vi "AMC QMH Template.vi"() -> ()   [LabVIEW 2017]
panel:
  out "Status":string
  in  "Process":bool
  in  "Exit":bool
  in  "State Variables":cluster{"CurrentFile":path}
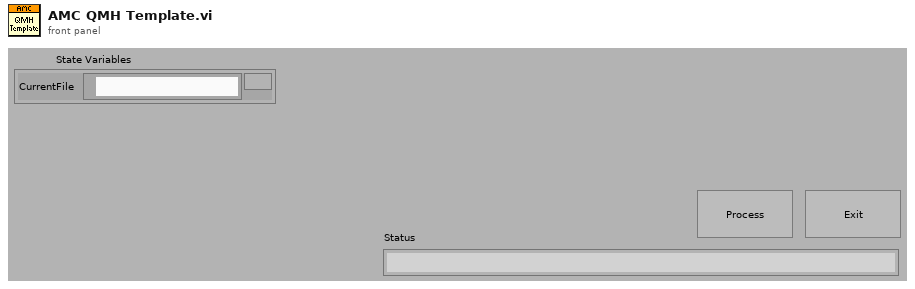
[diagram p1: front panel]
types:
  T1 = typedef "amc_Message Queue.ctl" = refnum<queue>
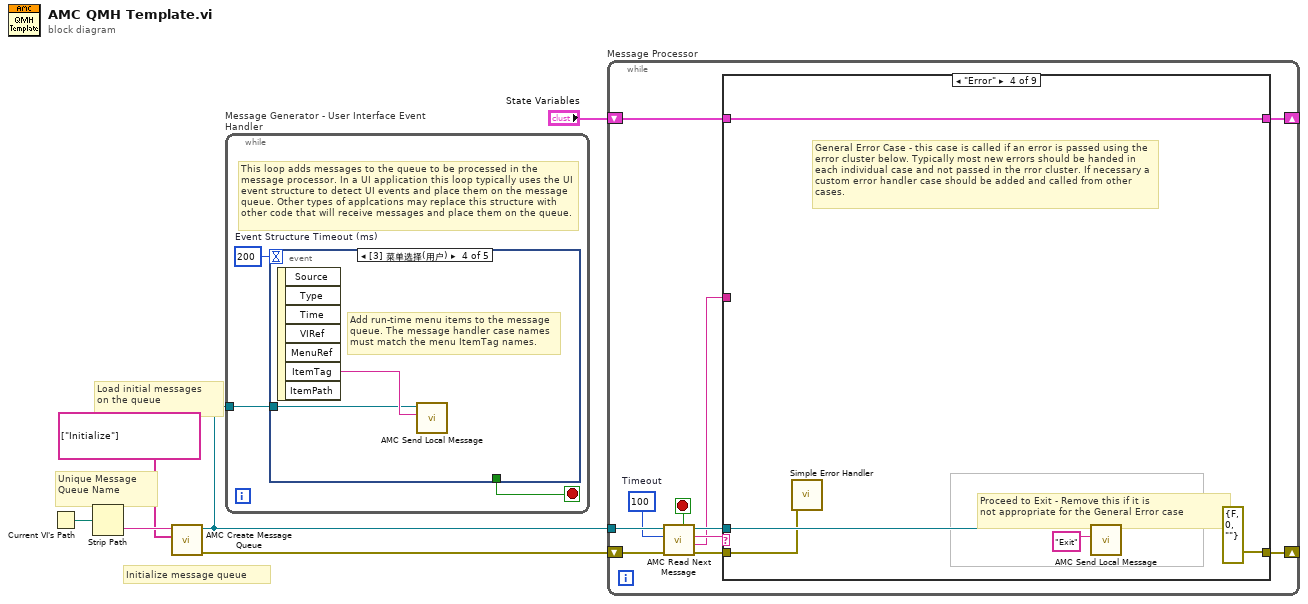
[diagram p0: block diagram]
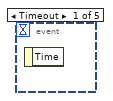
[diagram p2: hidden frame]
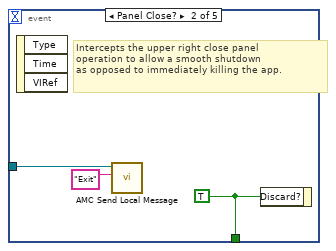
[diagram p3: hidden frame]
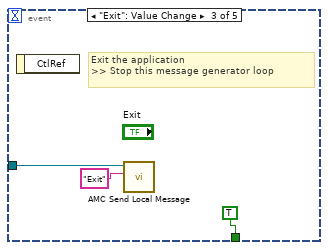
[diagram p4: hidden frame]
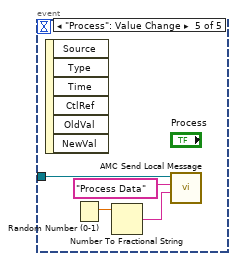
[diagram p5: hidden frame]
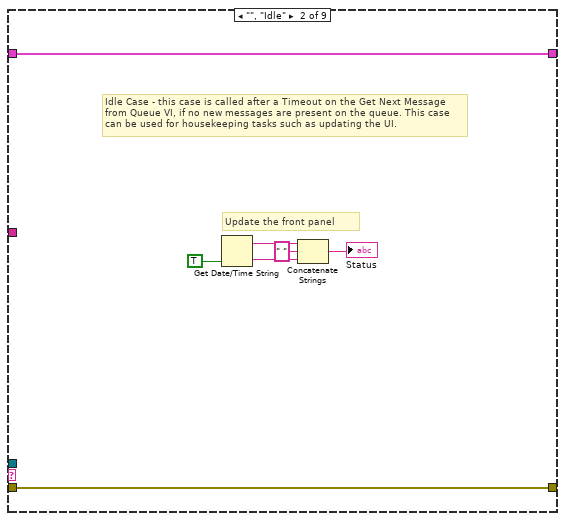
[diagram p7: hidden frame]
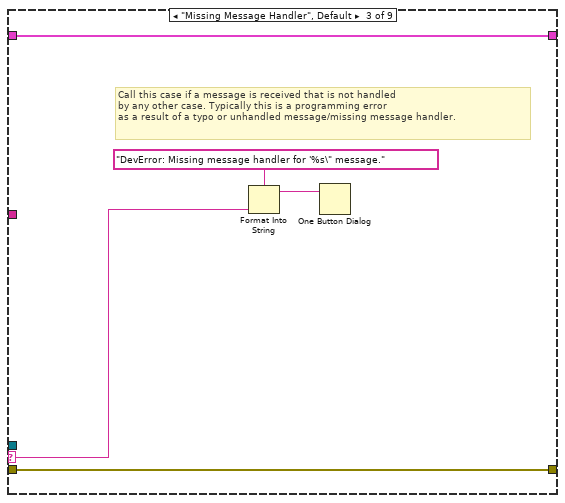
[diagram p8: hidden frame]
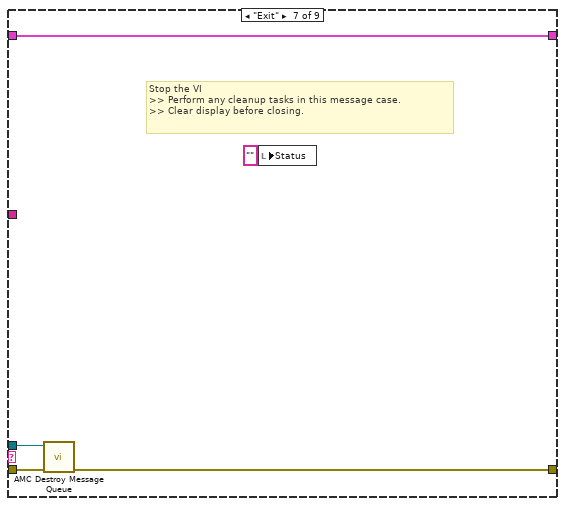
[diagram p11: hidden frame]
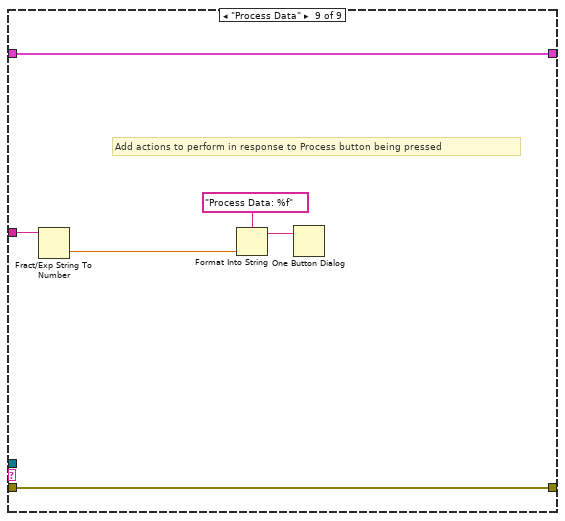
[diagram p13: hidden frame]
diagram:
  # "Initialize message queue"
  # "Unique Message\nQueue Name"
  # "Load initial messages\non the queue"
  n1 = Current VI's Path() -> (path=w6:path)
  n2 = Strip Path(path=w6) -> (name=w2:string)  [unwired: 1 out]
  n3 = call "AMC Create Message Queue.vi"("Initial Message Names"=string[] ["Initialize"], "Message Queue Name"=w2) -> ("error out"=w4:errorcluster, "Message Queue out"=w3:T1)  [unwired: 2 in, 6 out]
  n4 = while "Message Generator - User Interface Event Handler" {
    tunnel: w3 -> [w7]
    stop <- w8 stop-if-true
    w9 = 200  # Event Structure Timeout (ms)
    # "This loop adds messages to the queue to be processed in the message processor. In a UI application this loop typically uses the UI event structure to detect UI events and place them on the message queue. Other types of applcations may replace this structure with other code that will receive messages and place them on the queue."
    n5 = event shown="[3] 菜单选择(用户)" {
      selector: _ -> [_ _ _ _ _]
      dyn-events: _ -> [_ _ _ _ _]
      timeout: w9 -> [_ _ _ _ _]
      tunnel: [_ w12 TRUE ("Discard?") _ _] -> w8
      tunnel: w7 -> [_ w10 w13 w16 w21]
      event Timeout {
        n6 = event-data() -> ()  [unwired: 2 out]
      }
      event Panel Close? {
        w12 = TRUE ("Discard?")
        # "Intercepts the upper right close panel\noperation to allow a smooth shutdown\nas opposed to immediately killing the app."
        n7 = event-data() -> ()  [unwired: 4 out]
        n8 = call "AMC Send Local Message.vi"("Message Name"="Exit", "Message Queue in"=w10) -> ()  [unwired: 4 in, 6 out]
        n9 = event-data("Discard?"=w12) -> ()  [unwired: 1 in, 1 out]
      }
      event "Exit": Value Change {
        # "Exit the application\n>> Stop this message generator loop"
        n10 = event-data() -> ()  [unwired: 2 out]
        n11 = call "AMC Send Local Message.vi"("Message Name"="Exit", "Message Queue in"=w13) -> ()  [unwired: 4 in, 6 out]
      }
      event Menu Selection (User) {
        # "Add run-time menu items to the message\nqueue. The message handler case names must match the menu ItemTag names."
        n12 = event-data() -> ("ItemTag"=w17:string)  [unwired: 7 out]
        n13 = call "AMC Send Local Message.vi"("Message Name"=w17, "Message Queue in"=w16) -> ()  [unwired: 4 in, 6 out]
      }
      event "Process": Value Change {
        n14 = event-data() -> ()  [unwired: 7 out]
        n15 = Random Number (0-1)() -> (number: 0 to 1=w18:dbl)
        n16 = Number To Fractional String(number=w18) -> (F-format string=w19:string)  [unwired: 3 out]
        n17 = call "AMC Send Local Message.vi"("Message Value"=w19, "Message Name"="Process Data", "Message Queue in"=w21) -> ()  [unwired: 3 in, 6 out]
      }
    }
  }
  n18 = while "Message Processor" {
    shift-left: w4 -> [w26]
    shift-right: [w30] -> _
    tunnel: w3 -> [w27]
    shift-left: "State Variables" -> [w32]
    shift-right: [w31] -> _
    stop <- w29 stop-if-true
    w24 = 100  # Timeout
    n19 = call "AMC Read Next Message.vi"("error in (no error)"=w26, "timeout (1ms)"=w24, "Message Queue in"=w27) -> ("error out"=w25:errorcluster, "Message Value"=w22:string, "Message Name"=w23:string, "Message Queue out"=w28:T1, "Exit Process"=w29:bool)  [unwired: 1 in, 3 out]
    n20 = case shown="\"Error\"" w23 {
      selector: w23 -> [_ _ w44 _ _ _ _ _ _]
      tunnel: [w34 w41 w46 w51 w53 w55 w60 w62 w67] -> w31
      tunnel: w32 -> [w34 w41 w46 w51 w53 w55 w60 w62 w67]
      tunnel: w28 -> [_ _ _ w49 _ _ w57 _ _]
      tunnel: w25 -> [w33 w40 w45 w47 w52 w54 w58 w61 w68]
      tunnel: [w33 w40 w45 errorcluster {"status"=FALSE, "code"=0, "source"=""} ("error out") w52 w54 w56 w61 w68] -> w30
      tunnel: w22 -> [_ _ _ _ _ _ _ _ w66]
      frame "---------- Framework Operations ----------" {
        # "Dummy case to add a seperator in the Case Structure menu"
      }
      frame "", "Idle" {
        # "Update the front panel"
        # "Idle Case - this case is called after a Timeout on the Get Next Message from Queue VI, if no new messages are present on the queue. This case can be used for housekeeping tasks such as updating the UI."
        n21 = Get Date/Time String(want seconds? (F)=TRUE) -> (date string=w39:string, time string=w38:string)  [unwired: 2 out]
        n22 = Concatenate Strings(w39, " " ("string"), w38) -> (→"Status":string)
      }
      frame "Missing Message Handler", Default {
        # "Call this case if a message is received that is not handled \nby any other case. Typically this is a programming error\nas a result of a typo or unhandled message/missing message handler."
        n23 = Format Into String(format string="DevError: Missing message handler for '%s\" message." ("message"), w44) -> (resulting string=w42:string)  [unwired: 2 in, 1 out]
        n24 = One Button Dialog(message=w42) -> ()  [unwired: 2 out]
      }
      frame "Error" {
        # "Proceed to Exit - Remove this if it is\nnot appropriate for the General Error case"
        # "General Error Case - this case is called if an error is passed using the error cluster below. Typically most new errors should be handed in each individual case and not passed in the rror cluster. If necessary a custom error handler case should be added and called from other cases."
        n25 = call <vilib>:"Simple Error Handler.vi"("error in (no error)"=w47) -> ()  [unwired: 1 in, 8 out]
        n26 = call "AMC Send Local Message.vi"("Message Name"="Exit", "Message Queue in"=w49) -> ()  [unwired: 4 in, 6 out]
      }
      frame "---------- Generic Operations ----------" {
        # "Dummy case to add a seperator in the Case Structure menu"
      }
      frame "Initialize" {
        # "Initialize the state variables and user interface"
      }
      frame "Exit" {
        # "Stop the VI\n>> Perform any cleanup tasks in this message case.\n>> Clear display before closing."
        n27 = call "AMC Destroy Message Queue.vi"("error in (no error)"=w58, "Message Queue in"=w57) -> ("error out"=w56:errorcluster)  [unwired: 9 out]
        n28 = local write "Status"("" ("Status")) -> ()
      }
      frame "---------- Application Operations ----------" {
        # "Dummy case to add a seperator in the Case Structure menu"
      }
      frame "Process Data" {
        # "Add actions to perform in response to Process button being pressed"
        n29 = Fract/Exp String To Number(string=w66) -> (number=w65:dbl)  [unwired: 4 out]
        n30 = Format Into String(format string="Process Data: %f" ("message"), w65) -> (resulting string=w63:string)  [unwired: 2 in, 1 out]
        n31 = One Button Dialog(message=w63) -> ()  [unwired: 2 out]
      }
    }
  }
